vi "ChassisSystemEncoderControlledHolonomicDrive.vi"(0 "RobotDriveDevRef":T1={"DevStatus"={"status"=FALSE, "code"=0, "source"=""}, "Motors[]"=[], "Square Inputs"=FALSE, "Max Output"=1.0}, 1 "Robot Maximum Rate":dbl, 2 "Proportional Constant":dbl, 5 "X":dbl, 7 "Y":dbl, 9 "Rotation":dbl, 11 "error in (no error)":errorcluster, 12 "Encoder Readings":dbl[](array[numeric])) -> (4 "RobotDriveDevRef":T1={"DevStatus"={"status"=FALSE, "code"=0, "source"=""}, "Motors[]"=[], "Square Inputs"=FALSE, "Max Output"=1.0}, 8 "Motor Values":dbl[](array[numeric]), 15 "error out":errorcluster)   [LabVIEW 2014]
uses:
  <vilib>/Rock Robotics/WPI/RobotDrive/WPI_RobotDriveDevRef.ctl
  <vilib>/Rock Robotics/WPI/MotorControl/WPI_MotorControlDeviceRef.ctl
  <vilib>/Rock Robotics/WPI/MotorControl/WPI_MotorControlType.ctl
  <vilib>/Rock Robotics/SystemInterfaces/Typedef/FPGA_TypedefDigitalModule.ctl
  <vilib>/Rock Robotics/SystemInterfaces/DIO/FPGA_DIOPWMChannel.ctl
  <vilib>/Rock Robotics/WPI/PWM/WPI_PWMDeadband.ctl
  <vilib>/Rock Robotics/WPI/CAN/Jaguar/SubVIs/WPI_CANJaguar_ControlMode.ctl
  <vilib>/Rock Robotics/WPI/CAN/TalonSRX/WPI_CANTalonSRX_APIControlMode.ctl
  <vilib>/Rock Robotics/WPI/PWM/WPI_PWMTransform_ConPane.ctl
  <vilib>/Rock Robotics/SystemInterfaces/NetworkCommunication/NetComm_UsageReport_ResourceType.ctl
  <vilib>/Rock Robotics/WPI/RobotDrive/WPI_RobotDriveMotorSelectorEnum.ctl
  <vilib>/Rock Robotics/WPI/RobotDrive/WPI_RobotDriveSafetyCheck.vi
panel:
  in  "Gyro Angle":dbl
  # "**********************************************"
  # "Make sure this value is 0.046 every time"
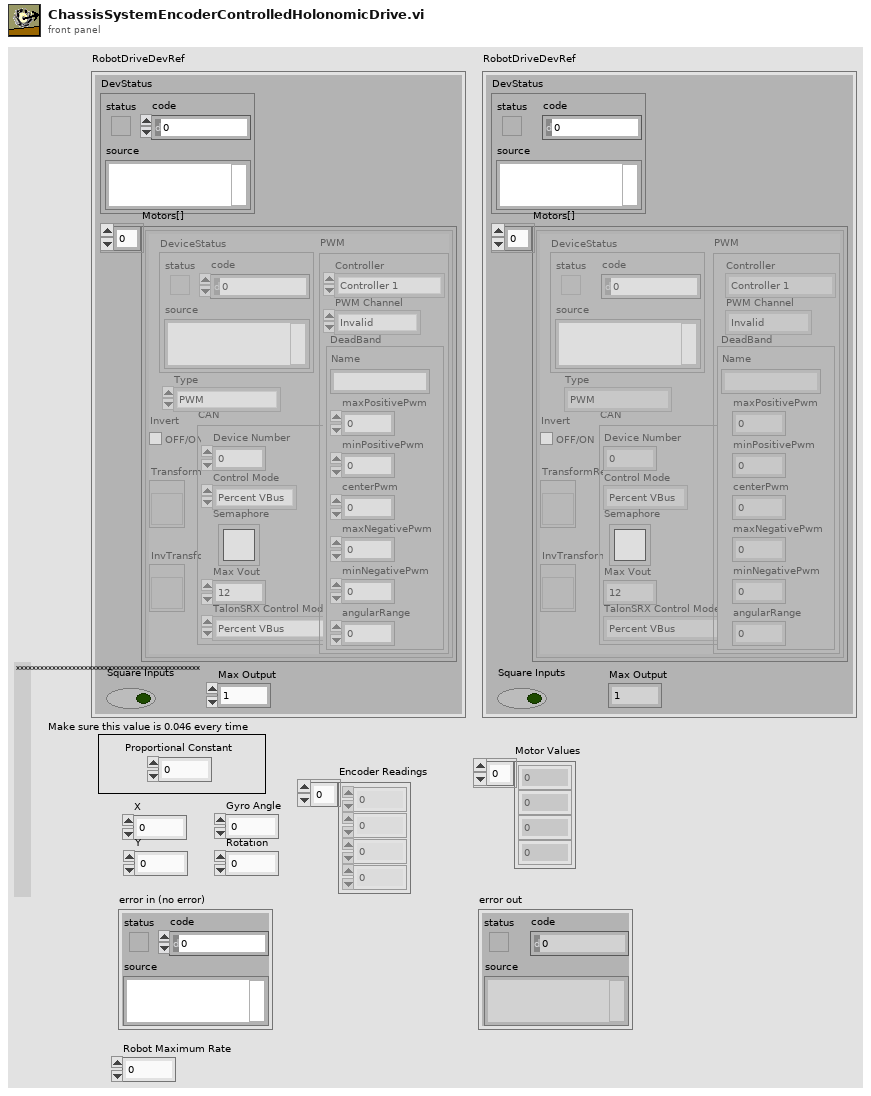
[diagram p1: front panel]
types:
  T1 = typedef "WPI_RobotDriveDevRef.ctl" = cluster{"DevStatus":errorcluster, "Motors[]":T2[], "Square Inputs":bool, "Max Output":dbl}
  T2 = typedef "WPI_MotorControlDeviceRef.ctl" = cluster{"DeviceStatus":errorcluster, "Type":T3, "PWM":cluster{"Controller":T4, "PWM Channel":T5, "DeadBand":T6}, "CAN":cluster{"Device Number":u8, "Control Mode":T7, "Semaphore":T8, "Max Vout":dbl, "TalonSRX Control Mode":T9}, "Invert":bool, "TransformRef":T10, "InvTransformRef":T10}
  T3 = typedef "WPI_MotorControlType.ctl" = enum16{"PWM", "CAN", "CANTalonSRX"}
  T4 = typedef "FPGA_TypedefDigitalModule.ctl" = enum16{"Controller 1"}
  T5 = typedef "FPGA_DIOPWMChannel.ctl" = enum8{"PWM 0", "PWM 1", "PWM 2", "PWM 3", "PWM 4", "PWM 5", "PWM 6", "PWM 7", "PWM 8", "PWM 9", "PWM MXP 0", "PWM MXP 1", "PWM MXP 2", "PWM MXP 3", "PWM MXP 4", "PWM MXP 5", "PWM MXP 6", "PWM MXP 7", "PWM MXP 8", "PWM MXP 9", "Invalid"}
  T6 = typedef "WPI_PWMDeadband.ctl" = cluster{"Name":string, "maxPositivePwm":i32, "minPositivePwm":i32, "centerPwm":i32, "maxNegativePwm":i32, "minNegativePwm":i32, "angularRange":u16}
  T7 = typedef "WPI_CANJaguar_ControlMode.ctl" = enum8{"Percent VBus", "Current", "Speed", "Position", "Voltage"}
  T8 = typedef "Semaphore RefNum" = refnum<k1>
  T9 = typedef "WPI_CANTalonSRX_APIControlMode.ctl" = enum8{"Percent VBus", "Speed", "Position", "Slave", "Unchanged / Invalid"}
  T10 = typedef "WPI_PWMTransform_ConPane.ctl" = refnum<vi>
  T11 = typedef "NetComm_UsageReport_ResourceType.ctl" = enum8{"Controller", "Module", "Language", "CANPlugin", "Accelerometer", "ADXL345", "AnalogChannel", "AnalogTrigger", "AnalogTriggerOutput", "CANJaguar", "Compressor", "Counter", "Dashboard", "DigitalInput", "DigitalOutput", "DriverStationCIO", "DriverStationEIO", "DriverStationLCD", "Encoder", "GearTooth", "Gyro", "I2C", "Framework", "Jaguar", "Joystick", "Kinect", "KinectStick", "PIDController", "Preferences", "PWM", "Relay", "RobotDrive", "SerialPort", "Servo", "Solenoid", "SPI", "Task", "Ultrasonic", "Victor", "Button", "Command", "AxisCamera", "PCVideoServer", "SmartDashboard", "Talon", "HiTechnicColorSensor", "HiTechnicAccel", "HiTechnicCompass", "SRF08", "AnalogOutput", "Victor SP", "Talon SRX", "CAN Talon SRX"}
  T12 = typedef "WPI_RobotDriveMotorSelectorEnum.ctl" = enum16{"Rear Left Motor", "Rear Right Motor", "Front Left Motor", "Front Right Motor"}
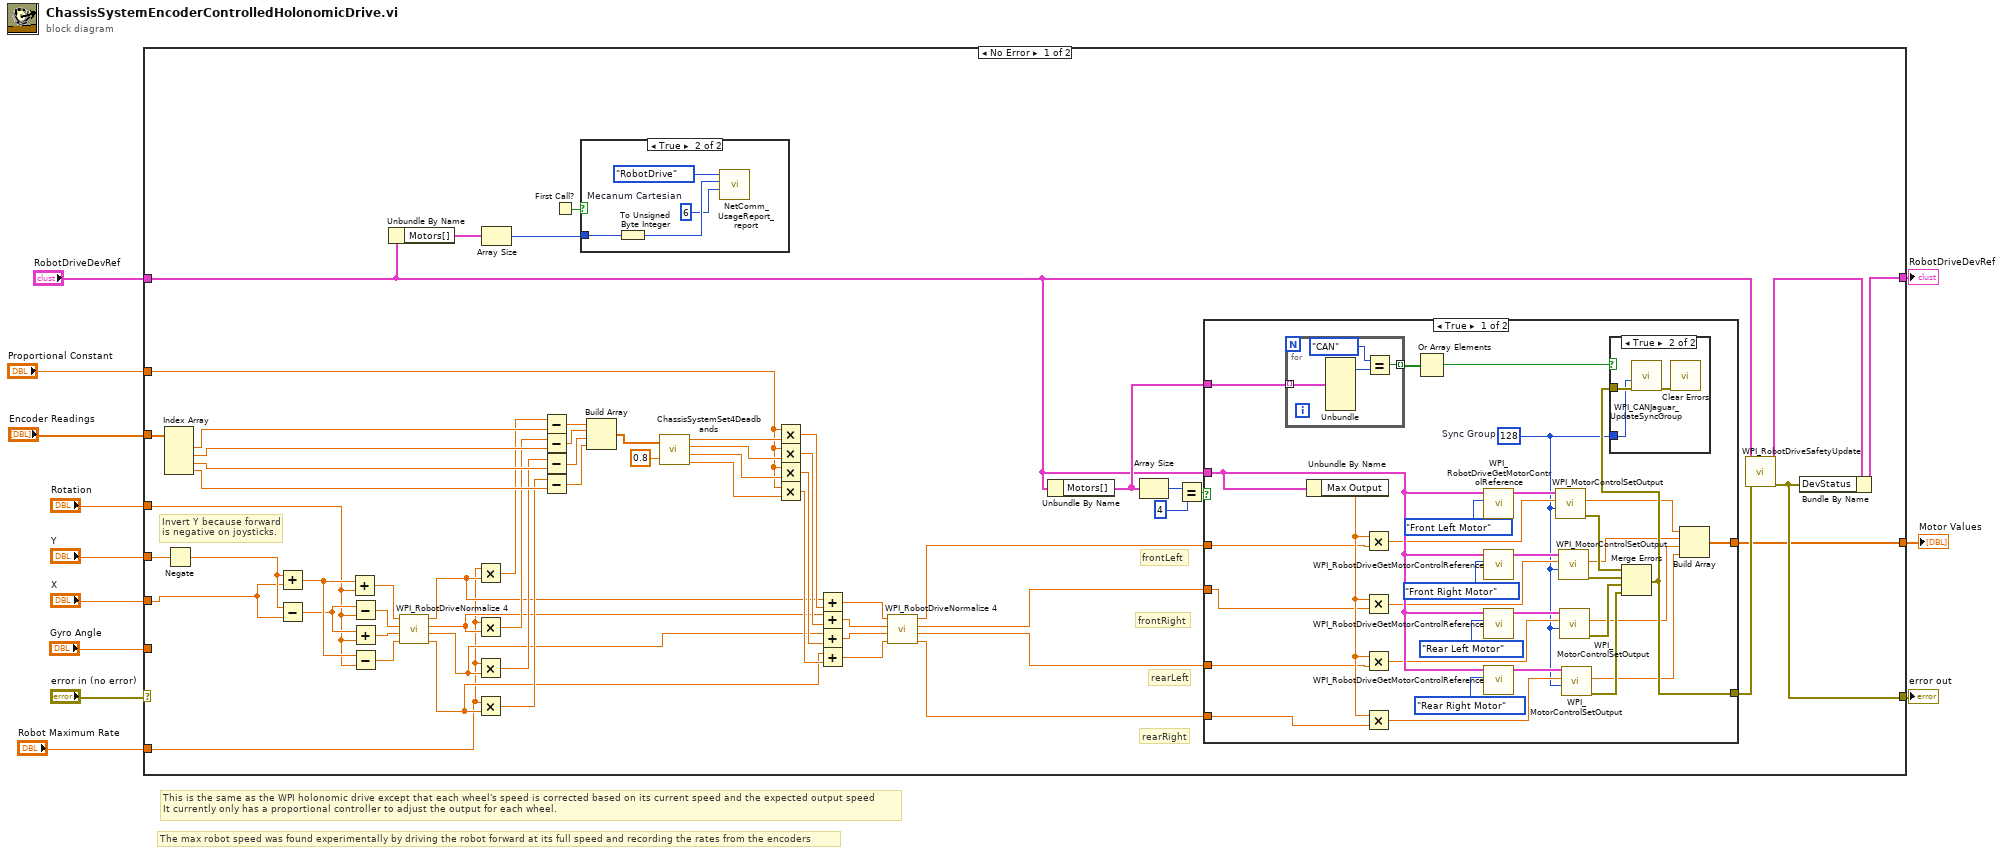
[diagram p0: block diagram]
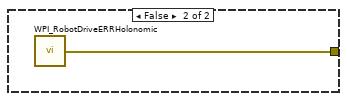
[diagram p4: hidden frame]
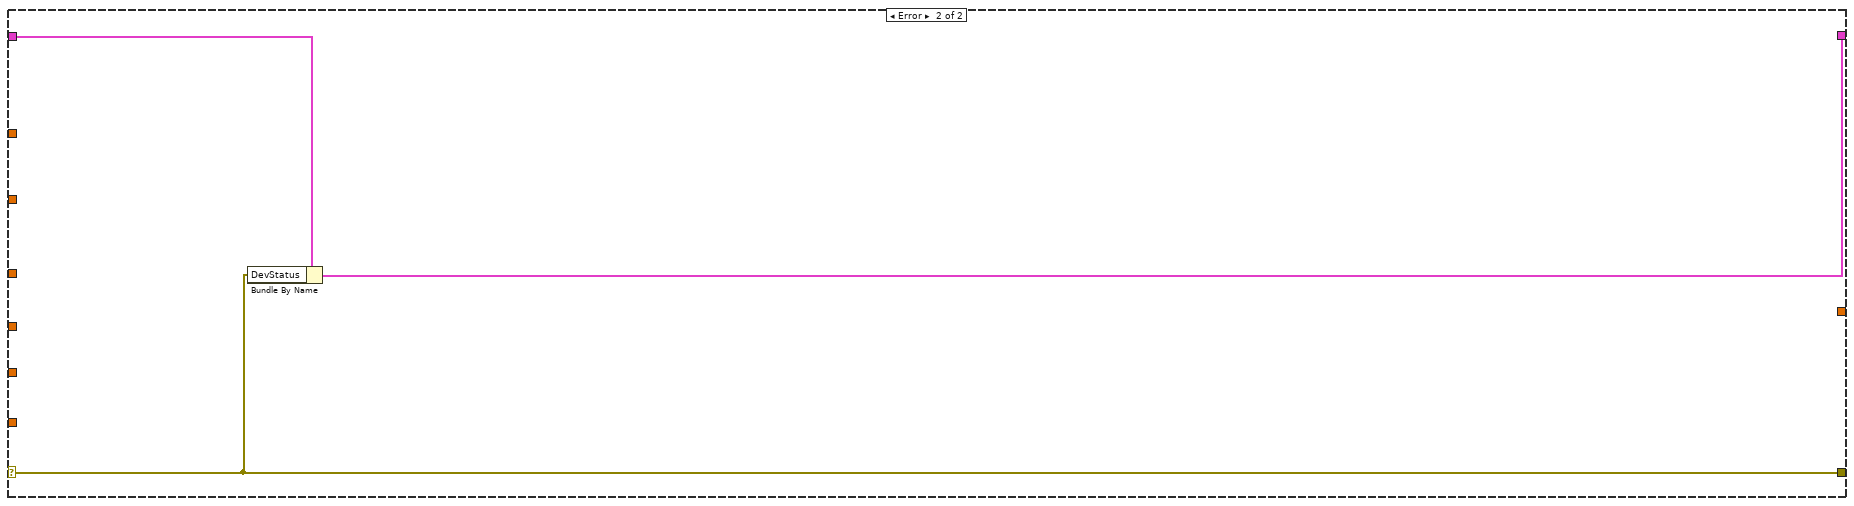
[diagram p5: hidden frame]
diagram:
  # "The max robot speed was found experimentally by driving the robot forward at its full speed and recording the rates from the encoders"
  # "This is the same as the WPI holonomic drive except that each wheel's speed is corrected based on its current speed and the expected output speed\nIt currently only has a proportional controller to adjust the output for each wheel."
  n1 = case shown="No Error" "error in (no error)" {
    selector: "error in (no error)" -> [_ w117]
    tunnel: "Y" -> [w61 _]
    tunnel: "X" -> [w50 _]
    tunnel: "RobotDriveDevRef" -> [w53 w119]
    tunnel: [w69 w118] -> w8
    tunnel: [w58 w117] -> w7
    tunnel: "Rotation" -> [w62 _]
    tunnel: "Gyro Angle" -> [_ _]
    tunnel: [w52 _] -> w4
    tunnel: "Proportional Constant" -> [w26 _]
    tunnel: "Encoder Readings" -> [w45 _]
    tunnel: "Robot Maximum Rate" -> [w13 _]
    frame No Error {
      # "Invert Y because forward is negative on joysticks."
      # "rearLeft"
      # "frontRight"
      # "rearRight"
      # "frontLeft"
      n2 = Index Array(array=w45) -> (element #1=w44:dbl, element #2=w43:dbl, element #3=w42:dbl, element #4=w41:dbl)  [unwired: 4 in]
      n3 = Negate(x=w61) -> (-x=w51:dbl)
      n4 = Add(x=w51, y=w50) -> (x+y=w67:dbl)
      n5 = Subtract(x=w51, y=w50) -> (x-y=w65:dbl)
      n6 = Add(x=w67, y=w62) -> (x+y=w63:dbl)
      n7 = Subtract(x=w65, y=w62) -> (x-y=w64:dbl)
      n8 = Add(x=w65, y=w62) -> (x+y=w66:dbl)
      n9 = Subtract(x=w67, y=w62) -> (x-y=w68:dbl)
      n10 = Unbundle By Name(w53) -> ("Motors[]"=w55:T2[])
      n11 = call <vilib>:"WPI_RobotDriveNormalize 4.vi"("D"=w68, "C"=w66, "B"=w64, "A"=w63) -> ("D'"=w14:dbl, "C'"=w17:dbl, "B'"=w16:dbl, "A'"=w15:dbl)
      n12 = Multiply(x=w13, y=w15) -> (x*y=w40:dbl)
      n13 = Multiply(x=w13, y=w16) -> (x*y=w39:dbl)
      n14 = Multiply(x=w13, y=w17) -> (x*y=w38:dbl)
      n15 = Multiply(x=w13, y=w14) -> (x*y=w37:dbl)
      n16 = Array Size(array=w55) -> (size(s)=w54:i32)
      n17 = Subtract(x=w40, y=w44) -> (x-y=w35:dbl)
      n18 = Subtract(x=w39, y=w43) -> (x-y=w34:dbl)
      n19 = Subtract(x=w38, y=w42) -> (x-y=w33:dbl)
      n20 = Subtract(x=w37, y=w41) -> (x-y=w32:dbl)
      n21 = First Call?() -> (First Call?: T/F=w56:bool)
      n22 = case shown="True" w56 {
        tunnel: w54 -> [_ w75]
        frame False {
        }
        frame True {
          w73 = u8 6  # Mecanum Cartesian
          n23 = To Unsigned Byte Integer(number=w75) -> (unsigned 8bit integer=w74:u8)
          n24 = call <vilib>:"NetComm_UsageReport_report.vi"("Context"=w73, "Instance Number"=w74, "Resource Type"=NetComm_UsageReport_ResourceType."RobotDrive") -> ()  [unwired: 9 in]
        }
      }
      n25 = Build Array(w35, w34, w33, w32) -> (w31:dbl[])
      n26 = call "ChassisSystemSet4Deadbands.vi"("Inputs"=w31, "Deadband"=0.8) -> ("Output 1"=w30:dbl, "Output 2"=w29:dbl, "Output 3"=w28:dbl, "Output 4"=w27:dbl)
      n27 = Multiply(x=w26, y=w30) -> (x*y=w18:dbl)
      n28 = Multiply(x=w26, y=w29) -> (x*y=w19:dbl)
      n29 = Multiply(x=w26, y=w28) -> (x*y=w20:dbl)
      n30 = Multiply(x=w26, y=w27) -> (x*y=w21:dbl)
      n31 = Add(x=w15, y=w18) -> (x+y=w23:dbl)
      n32 = Add(x=w16, y=w19) -> (x+y=w24:dbl)
      n33 = Add(x=w17, y=w20) -> (x+y=w25:dbl)
      n34 = Add(x=w14, y=w21) -> (x+y=w22:dbl)
      n35 = call <vilib>:"WPI_RobotDriveNormalize 4.vi"("D"=w22, "C"=w25, "B"=w24, "A"=w23) -> ("D'"=w46:dbl, "C'"=w47:dbl, "B'"=w48:dbl, "A'"=w49:dbl)
      n36 = Unbundle By Name(w53) -> ("Motors[]"=w57:T2[])
      n37 = Array Size(array=w57) -> (size(s)=w72:i32)
      n38 = Equal?(x=w72, y=4) -> (x = y?=w70:bool)
      n39 = case shown="True" w70 {
        tunnel: w53 -> [w100 _]
        tunnel: [w87 w116] -> w60
        tunnel: w57 -> [w88 _]
        tunnel: [w84 _] -> w52
        tunnel: w49 -> [w80 _]
        tunnel: w48 -> [w79 _]
        tunnel: w47 -> [w78 _]
        tunnel: w46 -> [w77 _]
        frame True {
          w86 = u8 128  # Sync Group
          n40 = for {
            tunnel: w88 -> [w112] mode=indexing
            tunnel: [w109] -> w89 mode=indexing
            n41 = Unbundle(w112) -> ("Type"=w111:T3)  [unwired: 6 out]
            n42 = Equal?(x=enum16{"PWM", "CAN"}."CAN" ("Type"), y=w111) -> (x = y?=w109:bool)
          }
          n43 = Unbundle By Name(w100) -> ("Max Output"=w95:dbl)
          n44 = Multiply(x=w95, y=w80) -> (x*y=w99:dbl)
          n45 = Multiply(x=w95, y=w79) -> (x*y=w98:dbl)
          n46 = Multiply(x=w95, y=w78) -> (x*y=w97:dbl)
          n47 = Multiply(x=w95, y=w77) -> (x*y=w96:dbl)
          n48 = Or Array Elements(Boolean array=w89) -> (logical OR=w90:bool)
          n49 = call <vilib>:"WPI_RobotDriveGetMotorControlReference.vi"("MotorIndex"=WPI_RobotDriveMotorSelectorEnum."Front Left Motor", "RobotDriveDevRef"=w100) -> ("MotorControlDeviceRef"=w108:T2)  [unwired: 9 out]
          n50 = call <vilib>:"WPI_RobotDriveGetMotorControlReference.vi"("MotorIndex"=WPI_RobotDriveMotorSelectorEnum."Front Right Motor", "RobotDriveDevRef"=w100) -> ("MotorControlDeviceRef"=w106:T2)  [unwired: 9 out]
          n51 = call <vilib>:"WPI_RobotDriveGetMotorControlReference.vi"("MotorIndex"=WPI_RobotDriveMotorSelectorEnum."Rear Left Motor", "RobotDriveDevRef"=w100) -> ("MotorControlDeviceRef"=w107:T2)  [unwired: 9 out]
          n52 = call <vilib>:"WPI_RobotDriveGetMotorControlReference.vi"("MotorIndex"=WPI_RobotDriveMotorSelectorEnum."Rear Right Motor", "RobotDriveDevRef"=w100) -> ("MotorControlDeviceRef"=w105:T2)  [unwired: 9 out]
          n53 = call <vilib>:"WPI_MotorControlSetOutput.vi"("Sync Group / Parameter Slot"=w86, "Output"=w99, "MotorControlDevRef"=w108) -> ("error out"=w91:errorcluster, "Motor Output"=w85:dbl)  [unwired: 2 in, 5 out]
          n54 = call <vilib>:"WPI_MotorControlSetOutput.vi"("Sync Group / Parameter Slot"=w86, "Output"=w98, "MotorControlDevRef"=w106) -> ("error out"=w92:errorcluster, "Motor Output"=w83:dbl)  [unwired: 2 in, 5 out]
          n55 = call <vilib>:"WPI_MotorControlSetOutput.vi"("Sync Group / Parameter Slot"=w86, "Output"=w97, "MotorControlDevRef"=w107) -> ("error out"=w93:errorcluster, "Motor Output"=w82:dbl)  [unwired: 2 in, 5 out]
          n56 = call <vilib>:"WPI_MotorControlSetOutput.vi"("Sync Group / Parameter Slot"=w86, "Output"=w96, "MotorControlDevRef"=w105) -> ("error out"=w94:errorcluster, "Motor Output"=w81:dbl)  [unwired: 2 in, 5 out]
          n57 = Merge Errors(w91, w92, w93, w94) -> (w87:errorcluster)
          n58 = case shown="True" w90 {
            tunnel: w87 -> [_ w114]
            tunnel: w86 -> [_ w113]
            frame False {
            }
            frame True {
              n59 = call <vilib>:"WPI_CANJaguar_UpdateSyncGroup.vi"("error in (no error)"=w114, "Sync Group"=w113) -> ("error out"=w115:errorcluster)  [unwired: 9 out]
              n60 = call <vilib>:"Clear Errors.vi"("error in (no error)"=w115) -> ()  [unwired: 1 in, 6 out]
            }
          }
          n61 = Build Array(w85, w83, w82, w81) -> (w84:dbl[])
        }
        frame False {
          n62 = call <vilib>:"WPI_RobotDriveERRHolonomic.vi"() -> ("error out"=w116:errorcluster)
        }
      }
      n63 = call <vilib>:"WPI_RobotDriveSafetyUpdate.vi"("error in (no error)"=w60, "RobotDriveDevRef"=w53) -> ("error out"=w58:errorcluster, "RobotDriveDevRef"=w59:T1)  [unwired: 8 out]
      n64 = Bundle By Name(cluster=w59, "DevStatus"=w58) -> (w69:T1)
    }
    frame Error {
      n65 = Bundle By Name(cluster=w119, "DevStatus"=w117) -> (w118:T1)
    }
  }
  "error out" <- w7
  "RobotDriveDevRef" <- w8
  "Motor Values" <- w4
